vi "Drive Controller.vi"(8 "error in":errorcluster) -> ()   [LabVIEW 2020]
doc: "This VI executes continuously carrying out the current operation and responding to updates or new operation requests. It will often contain the timing or control code that is difficult to place directly in TeleOp. This VI generally opens all sensors and motors and isolates the rest of the robot code from knowing implementation details of how the operations are carried out."
uses:
  <vilib>/Rock Robotics/WPI/Framework/Completion Status.ctl
  Drive Setpoints.ctl
  Drive Operations.ctl
  <vilib>/Rock Robotics/WPI/SafetyOutput/WPI_SafetyOutputConfigMenu.ctl
  <vilib>/Rock Robotics/WPI/ThirdParty/REV Robotics/REVLib/Typedef/Spark MAX Idle Mode.ctl
  <vilib>/Rock Robotics/WPI/RobotDrive/WPI_RobotDriveOpen2MotorWithExistingMotors.vi
  <vilib>/Rock Robotics/Network Tables/NT Write Numeric Array.vi
  <vilib>/Rock Robotics/WPI/ThirdParty/REV Robotics/REVLib/Typedef/Spark MAX Motor Type.ctl
panel:
  in  "Interactive Values":T1
  in  "Buttons":cluster{"Execute Cmd":bool, "Abort Cmd":bool}
  out "Command Timing":cluster{"Start Time (ms)":u32, "Iterations":i32}
  out "Status":T3
  out "Setpoints":T4(graph)
  out "Current\nCmd":string
  # "Tip: The graph shows the motor setpoints. It may also be helpful to observe inputs and sensor values.\nYou may also want to display tuning or debugging controls."
  # "Interactive Command: You may fill in the settings for a command\nand schedule it with the Execute button. You can observe and abort\nany command while fine tuning the code for the controller."
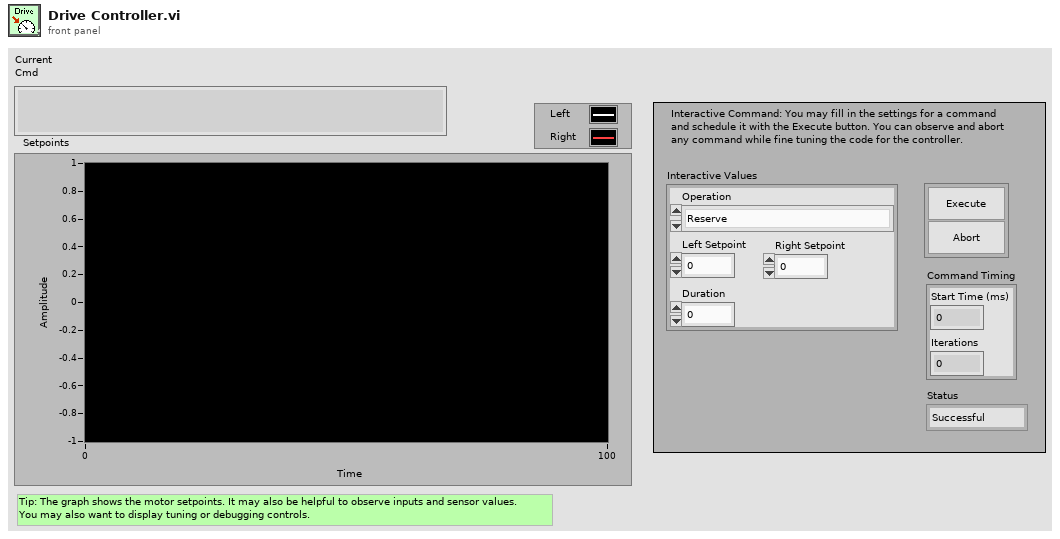
[diagram p1: front panel]
types:
  T1 = typedef "Drive Setpoints.ctl" = cluster{"Operation":T2, "Left Setpoint":dbl, "Right Setpoint":dbl, "Duration":dbl}
  T2 = typedef "Drive Operations.ctl" = enum16{"Reserve", "Read Current", "Immediate", "Drive for Time", "Drive for Distance"}
  T3 = typedef "Completion Status.ctl" = enum16{"Successful", "Aborted", "Incomplete"}
  T4 = cluster{"Left Setpoint":dbl, "Right Setpoint":dbl}
  T5 = typedef "WPI_SafetyOutputConfigMenu.ctl" = enum16{"Enable", "Disable"}
  T6 = typedef "Spark MAX Idle Mode.ctl" = enum16{"Coast", "Brake"}
  T7 = typedef "WPI_MotorControlDeviceRef.ctl" = cluster{"DeviceStatus":errorcluster, "Type":T8, "PWM":cluster{"PWM Channel":T9, "DeadBand":T10}, "CAN":cluster{"Device Number":u8, "SetOutput VI Ref":variant, "GetOutput VI Ref":variant, "Enable VI Ref":variant, "Disable VI Ref":variant, "Data":variant}, "Invert":bool, "DIO PWM":cluster{"PWM \"Enable\" Channel":T9, "DIOChannel":T11, "PWM Rate":dbl}}
  T8 = typedef "WPI_MotorControlType.ctl" = enum16{"PWM", "CAN", "DIO PWM"}
  T9 = typedef "FPGA_DIOPWMChannel.ctl" = enum8{"PWM 0", "PWM 1", "PWM 2", "PWM 3", "PWM 4", "PWM 5", "PWM 6", "PWM 7", "PWM 8", "PWM 9", "PWM MXP 0", "PWM MXP 1", "PWM MXP 2", "PWM MXP 3", "PWM MXP 4", "PWM MXP 5", "PWM MXP 6", "PWM MXP 7", "PWM MXP 8", "PWM MXP 9", "Invalid"}
  T10 = typedef "WPI_PWMDeadband.ctl" = cluster{"Name":string, "maxPositivePwm":i32, "minPositivePwm":i32, "centerPwm":i32, "maxNegativePwm":i32, "minNegativePwm":i32, "angularRange":u16}
  T11 = typedef "FPGA_DIOChannel.ctl" = enum8{"DIO 0", "DIO 1", "DIO 2", "DIO 3", "DIO 4", "DIO 5", "DIO 6", "DIO 7", "DIO 8", "DIO 9", "DIO MXP 0", "DIO MXP 1", "DIO MXP 2", "DIO MXP 3", "DIO MXP 4", "DIO MXP 5", "DIO MXP 6", "DIO MXP 7", "DIO MXP 8", "DIO MXP 9", "DIO MXP 10", "DIO MXP 11", "DIO MXP 12", "DIO MXP 13", "DIO MXP 14", "DIO MXP 15", "SPI Port CS1", "SPI Port CS2", "SPI Port CS3", "SPI Port MISO", "SPI Port MOSI", "Invalid"}
  T12 = typedef "Spark MAX Motor Type.ctl" = enum16{"Brushed", "Brushless"}
  T13 = typedef "WPI_RobotDriveDevRef.ctl" = cluster{"DevStatus":errorcluster, "Motors[]":T7[], "Square Inputs":bool, "Max Output":dbl}
  T14 = typedef "Command Status Info.ctl" = cluster{"Name":string, "Status":T3, "notifier out":T15}
  T15 = typedef "Completion Notifier.ctl" = refnum<notifier>
  T16 = cluster{"SubSystem Data":T1, cluster{"Start Time (ms)":u32, "Iterations":i32}, cluster{"Command Info":T14, "Description":string, "Default Command":T1, "queue out":refnum<queue>, "Subsystem Name":string}}
  T17 = cluster{"SubSystem Data":T1, cluster{"Start Time (ms)":u32, "Iterations":i32}, "Default Command Arguments":cluster{"Command Info":T14, "Description":string, "Default Command":T1, "queue out":refnum<queue>, "Subsystem Name":string}}
  T18 = cluster{"Don't move motors while reserved":dbl, "Don't move motors while reserved":dbl}
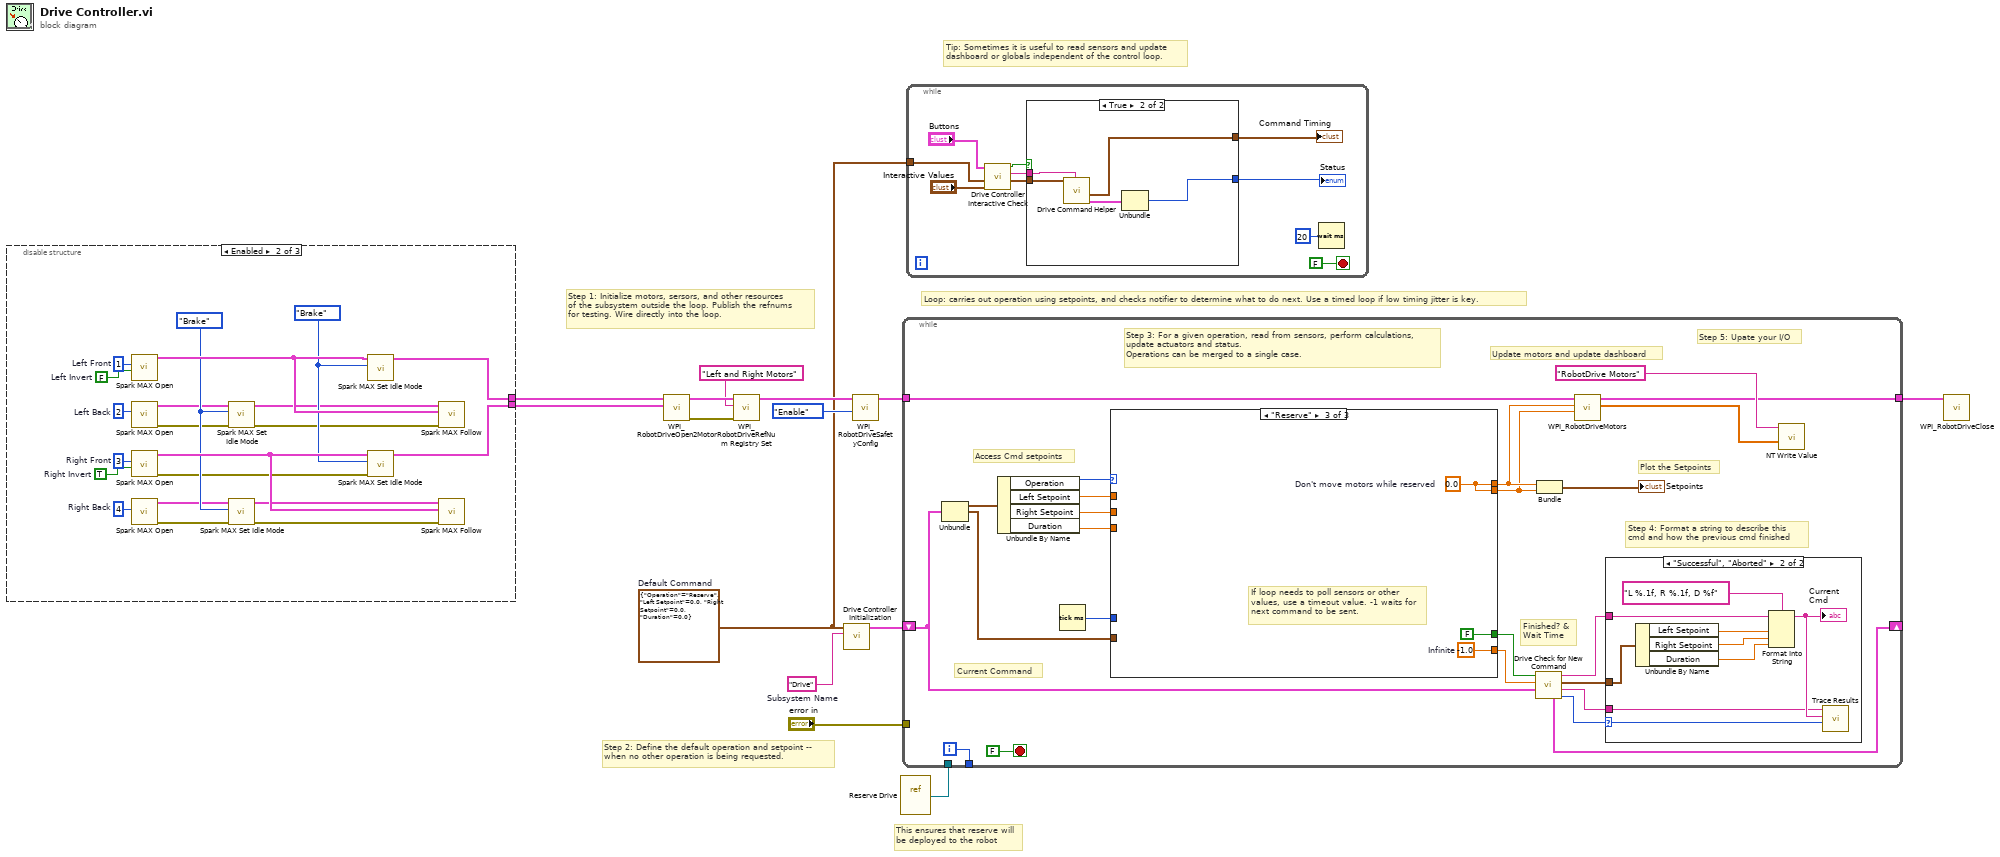
[diagram p0: block diagram]
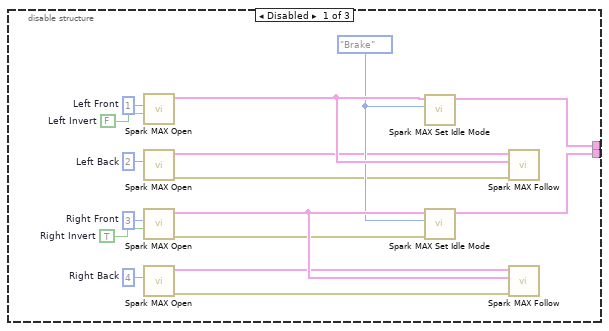
[diagram p2: hidden frame]
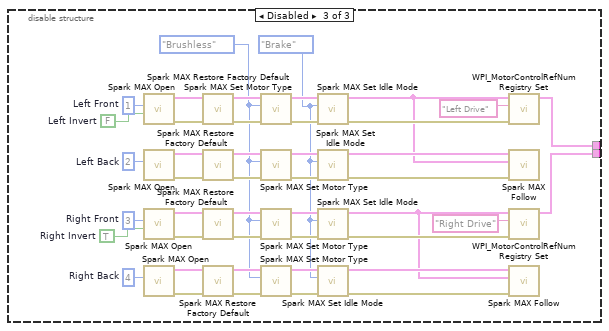
[diagram p3: hidden frame]
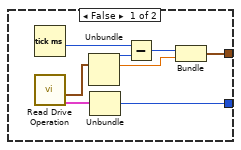
[diagram p4: hidden frame]
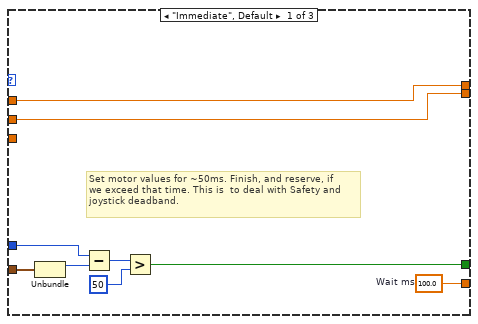
[diagram p6: hidden frame]
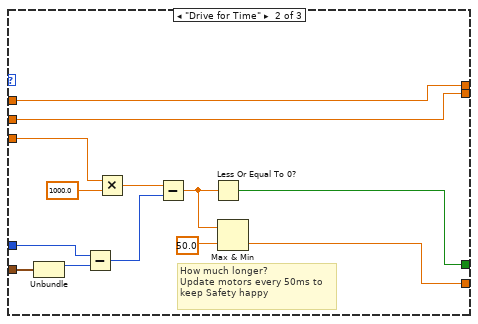
[diagram p7: hidden frame]
diagram:
  w4 = T1 {"Operation"=enum."Reserve", "Left Setpoint"=0.0, "Right Setpoint"=0.0, "Duration"=0.0}  # Default Command
  w14 = "Drive"  # Subsystem Name
  # "This ensures that reserve will\nbe deployed to the robot"
  # "Tip: Sometimes it is useful to read sensors and update\ndashboard or globals independent of the control loop."
  # "Step 2: Define the default operation and setpoint --\nwhen no other operation is being requested."
  # "Step 1: Initialize motors, sersors, and other resources\nof the subsystem outside the loop. Publish the refnums\nfor testing. Wire directly into the loop."
  # "Loop: carries out operation using setpoints, and checks notifier to determine what to do next. Use a timed loop if low timing jitter is key."
  n1 = disable-structure shown="Enabled" {
    disable-tunnel: [w23 w44 w55] -> w3
    disable-tunnel: [w21 w42 w54] -> w2
    frame Disabled {
      w20 = Spark_MAX_Idle_Mode."Brake" ("Idle Mode")
      w25 = u8 4  # Right Back
      w26 = u8 3  # Right Front
      w27 = u8 2  # Left Back
      w28 = u8 1  # Left Front
      w29 = TRUE  # Right Invert
      w30 = FALSE  # Left Invert
      n2 = call <vilib>:"Spark MAX Open.vi"("Invert"=w30, "Device Number"=w28) -> ("MotorControlDeviceRef"=w24:T7)  [unwired: 8 in, 1 out]
      n3 = call <vilib>:"Spark MAX Open.vi"("Device Number"=w27) -> ("error out"=w18:errorcluster, "MotorControlDeviceRef"=w19:T7)  [unwired: 9 in]
      n4 = call <vilib>:"Spark MAX Open.vi"("Invert"=w29, "Device Number"=w26) -> ("error out"=w17:errorcluster, "MotorControlDeviceRef"=w22:T7)  [unwired: 8 in]
      n5 = call <vilib>:"Spark MAX Open.vi"("Device Number"=w25) -> ("error out"=w15:errorcluster, "MotorControlDeviceRef"=w16:T7)  [unwired: 9 in]
      n6 = call <vilib>:"Spark MAX Set Idle Mode.vi"("Idle Mode"=w20, "MotorControlDeviceRef in"=w24) -> ("MotorControlDeviceRef out"=w23:T7)  [unwired: 8 in, 1 out]
      n7 = call <vilib>:"Spark MAX Set Idle Mode.vi"("error in (no error)"=w17, "Idle Mode"=w20, "MotorControlDeviceRef in"=w22) -> ("MotorControlDeviceRef out"=w21:T7)  [unwired: 7 in, 1 out]
      n8 = call <vilib>:"Spark MAX Follow.vi"("error in (no error)"=w18, "Master Controller"=w24, "MotorControlDeviceRef"=w19) -> ()  [unwired: 7 in, 2 out]
      n9 = call <vilib>:"Spark MAX Follow.vi"("error in (no error)"=w15, "Master Controller"=w22, "MotorControlDeviceRef"=w16) -> ()  [unwired: 7 in, 2 out]
    }
    frame Enabled {
      w40 = Spark_MAX_Idle_Mode."Brake" ("Idle Mode")
      w41 = Spark_MAX_Idle_Mode."Brake" ("Idle Mode")
      w46 = u8 4  # Right Back
      w47 = u8 3  # Right Front
      w48 = u8 2  # Left Back
      w49 = u8 1  # Left Front
      w50 = TRUE  # Right Invert
      w51 = FALSE  # Left Invert
      n10 = call <vilib>:"Spark MAX Open.vi"("Invert"=w51, "Device Number"=w49) -> ("MotorControlDeviceRef"=w45:T7)  [unwired: 8 in, 1 out]
      n11 = call <vilib>:"Spark MAX Open.vi"("Device Number"=w48) -> ("error out"=w37:errorcluster, "MotorControlDeviceRef"=w39:T7)  [unwired: 9 in]
      n12 = call <vilib>:"Spark MAX Open.vi"("Invert"=w50, "Device Number"=w47) -> ("error out"=w35:errorcluster, "MotorControlDeviceRef"=w43:T7)  [unwired: 8 in]
      n13 = call <vilib>:"Spark MAX Open.vi"("Device Number"=w46) -> ("error out"=w32:errorcluster, "MotorControlDeviceRef"=w34:T7)  [unwired: 9 in]
      n14 = call <vilib>:"Spark MAX Set Idle Mode.vi"("error in (no error)"=w37, "Idle Mode"=w40, "MotorControlDeviceRef in"=w39) -> ("error out"=w36:errorcluster, "MotorControlDeviceRef out"=w38:T7)  [unwired: 7 in]
      n15 = call <vilib>:"Spark MAX Set Idle Mode.vi"("error in (no error)"=w32, "Idle Mode"=w40, "MotorControlDeviceRef in"=w34) -> ("error out"=w31:errorcluster, "MotorControlDeviceRef out"=w33:T7)  [unwired: 7 in]
      n16 = call <vilib>:"Spark MAX Set Idle Mode.vi"("Idle Mode"=w41, "MotorControlDeviceRef in"=w45) -> ("MotorControlDeviceRef out"=w44:T7)  [unwired: 8 in, 1 out]
      n17 = call <vilib>:"Spark MAX Set Idle Mode.vi"("error in (no error)"=w35, "Idle Mode"=w41, "MotorControlDeviceRef in"=w43) -> ("MotorControlDeviceRef out"=w42:T7)  [unwired: 7 in, 1 out]
      n18 = call <vilib>:"Spark MAX Follow.vi"("error in (no error)"=w36, "Master Controller"=w45, "MotorControlDeviceRef"=w38) -> ()  [unwired: 7 in, 2 out]
      n19 = call <vilib>:"Spark MAX Follow.vi"("error in (no error)"=w31, "Master Controller"=w43, "MotorControlDeviceRef"=w33) -> ()  [unwired: 7 in, 2 out]
    }
    frame Disabled {
      w52 = Spark_MAX_Idle_Mode."Brake" ("Idle Mode")
      w53 = Spark_MAX_Motor_Type."Brushless" ("Motor Type")
      w62 = u8 4  # Right Back
      w63 = u8 3  # Right Front
      w64 = u8 2  # Left Back
      w65 = u8 1  # Left Front
      w66 = TRUE  # Right Invert
      w67 = FALSE  # Left Invert
      n20 = call <vilib>:"Spark MAX Open.vi"("Invert"=w67, "Device Number"=w65) -> ("error out"=w95:errorcluster, "MotorControlDeviceRef"=w94:T7)  [unwired: 8 in]
      n21 = call <vilib>:"Spark MAX Open.vi"("Device Number"=w64) -> ("error out"=w84:errorcluster, "MotorControlDeviceRef"=w85:T7)  [unwired: 9 in]
      n22 = call <vilib>:"Spark MAX Open.vi"("Invert"=w66, "Device Number"=w63) -> ("error out"=w78:errorcluster, "MotorControlDeviceRef"=w79:T7)  [unwired: 8 in]
      n23 = call <vilib>:"Spark MAX Open.vi"("Device Number"=w62) -> ("error out"=w73:errorcluster, "MotorControlDeviceRef"=w72:T7)  [unwired: 9 in]
      n24 = call <vilib>:"Spark MAX Restore Factory Default.vi"("error in"=w95, "MotorControlDeviceRef"=w94) -> ("error out"=w93:errorcluster, "MotorControlDeviceRef"=w92:T7)  [unwired: 8 in]
      n25 = call <vilib>:"Spark MAX Restore Factory Default.vi"("error in"=w84, "MotorControlDeviceRef"=w85) -> ("error out"=w86:errorcluster, "MotorControlDeviceRef"=w87:T7)  [unwired: 8 in]
      n26 = call <vilib>:"Spark MAX Restore Factory Default.vi"("error in"=w78, "MotorControlDeviceRef"=w79) -> ("error out"=w80:errorcluster, "MotorControlDeviceRef"=w81:T7)  [unwired: 8 in]
      n27 = call <vilib>:"Spark MAX Restore Factory Default.vi"("error in"=w73, "MotorControlDeviceRef"=w72) -> ("error out"=w71:errorcluster, "MotorControlDeviceRef"=w70:T7)  [unwired: 8 in]
      n28 = call <vilib>:"Spark MAX Set Motor Type.vi"("error in (no error)"=w93, "Motor Type"=w53, "MotorControlDevRef"=w92) -> ("error out"=w91:errorcluster, "MotorControlDeviceRef"=w90:T7)  [unwired: 7 in]
      n29 = call <vilib>:"Spark MAX Set Motor Type.vi"("error in (no error)"=w86, "Motor Type"=w53, "MotorControlDevRef"=w87) -> ("error out"=w88:errorcluster, "MotorControlDeviceRef"=w89:T7)  [unwired: 7 in]
      n30 = call <vilib>:"Spark MAX Set Motor Type.vi"("error in (no error)"=w80, "Motor Type"=w53, "MotorControlDevRef"=w81) -> ("error out"=w82:errorcluster, "MotorControlDeviceRef"=w83:T7)  [unwired: 7 in]
      n31 = call <vilib>:"Spark MAX Set Motor Type.vi"("error in (no error)"=w71, "Motor Type"=w53, "MotorControlDevRef"=w70) -> ("error out"=w69:errorcluster, "MotorControlDeviceRef"=w68:T7)  [unwired: 7 in]
      n32 = call <vilib>:"Spark MAX Set Idle Mode.vi"("error in (no error)"=w91, "Idle Mode"=w52, "MotorControlDeviceRef in"=w90) -> ("error out"=w61:errorcluster, "MotorControlDeviceRef out"=w59:T7)  [unwired: 7 in]
      n33 = call <vilib>:"Spark MAX Set Idle Mode.vi"("error in (no error)"=w88, "Idle Mode"=w52, "MotorControlDeviceRef in"=w89) -> ("error out"=w77:errorcluster, "MotorControlDeviceRef out"=w76:T7)  [unwired: 7 in]
      n34 = call <vilib>:"Spark MAX Set Idle Mode.vi"("error in (no error)"=w82, "Idle Mode"=w52, "MotorControlDeviceRef in"=w83) -> ("error out"=w60:errorcluster, "MotorControlDeviceRef out"=w58:T7)  [unwired: 7 in]
      n35 = call <vilib>:"Spark MAX Set Idle Mode.vi"("error in (no error)"=w69, "Idle Mode"=w52, "MotorControlDeviceRef in"=w68) -> ("error out"=w74:errorcluster, "MotorControlDeviceRef out"=w75:T7)  [unwired: 7 in]
      n36 = call <vilib>:"WPI_MotorControlRefNum Registry Set.vi"("error in (no error)"=w61, "refnum name"="Left Drive", "MotorControlDevRef"=w59) -> ("MotorControlDevRef"=w55:T7)  [unwired: 7 in, 1 out]
      n37 = call <vilib>:"Spark MAX Follow.vi"("error in (no error)"=w77, "Master Controller"=w59, "MotorControlDeviceRef"=w76) -> ()  [unwired: 7 in, 2 out]
      n38 = call <vilib>:"WPI_MotorControlRefNum Registry Set.vi"("error in (no error)"=w60, "refnum name"="Right Drive", "MotorControlDevRef"=w58) -> ("MotorControlDevRef"=w54:T7)  [unwired: 7 in, 1 out]
      n39 = call <vilib>:"Spark MAX Follow.vi"("error in (no error)"=w74, "Master Controller"=w58, "MotorControlDeviceRef"=w75) -> ()  [unwired: 7 in, 2 out]
    }
  }
  n40 = call-poly <vilib>:"WPI_RobotDriveOpen2Motor.vi"("Right Motor Dev Ref"=w2, "Left Motor Dev Ref"=w3) -> ("error out"=w11:errorcluster, "RobotDriveDevRef"=w13:T13)  [unwired: 3 in, 5 out]
  n41 = call <vilib>:"WPI_RobotDriveRefNum Registry Set.vi"("error in (no error)"=w11, "refnum name"="Left and Right Motors", "RobotDriveDevRef"=w13) -> ("RobotDriveDevRef"=w10:T13)  [unwired: 1 in, 7 out]
  n42 = call "Drive Controller Initialization.vi"("Subsystem Name"=w14, "Default Command"=w4) -> ("Current Command"=w6:T16)  [unwired: 9 in]
  n43 = call <vilib>:"WPI_RobotDriveSafetyConfig.vi"("mode"=WPI_SafetyOutputConfigMenu."Enable", "RobotDriveDevRef"=w10) -> ("RobotDriveDevRef"=w8:T13)  [unwired: 8 in, 1 out]
  n44 = vi-ref "Reserve Drive.vi"() -> (w5:refnum<vi>)
  n45 = while {
    shift-right: [w106] -> _
    shift-left: w6 -> [w99]
    tunnel: [w118] -> _
    tunnel: w8 -> [w114]
    tunnel: "error in" -> [_]
    tunnel: w5 -> [_]
    tunnel: [w96] -> w1
    i -> [w118]
    stop <- FALSE stop-if-true
    # "Step 5: Upate your I/O"
    # "Step 4: Format a string to describe this\ncmd and how the previous cmd finished"
    # "Current Command"
    # "Update motors and update dashboard"
    # "Plot the Setpoints"
    # "Access Cmd setpoints"
    # "Finished? &\nWait Time"
    # "Step 3: For a given operation, read from sensors, perform calculations,\nupdate actuators and status.\nOperations can be merged to a single case."
    n46 = Unbundle(w99) -> ("SubSystem Data"=w113:T1, w100:cluster{"Start Time (ms)":u32, "Iterations":i32})  [unwired: 1 out]
    n47 = Unbundle By Name(w113) -> ("Operation"=w112:T2, "Left Setpoint"=w111:dbl, "Right Setpoint"=w110:dbl, "Duration"=w109:dbl)
    n48 = Tick Count (ms)() -> (millisecond timer value=w108:u32)
    n49 = case shown="\"Reserve\"" w112 {
      tunnel: [w137 w138 w153] -> w105
      tunnel: [w130 w145 FALSE ("ignore previous (F)")] -> w104
      tunnel: w100 -> [w129 w147 _]
      tunnel: [w136 w144 w151] -> w116
      tunnel: [w135 w143 w151] -> w115
      tunnel: w111 -> [w136 w144 _]
      tunnel: w110 -> [w135 w143 _]
      tunnel: w109 -> [_ w142 _]
      tunnel: w108 -> [w131 w141 _]
      frame "Immediate", Default {
        w137 = 100.0  # Wait ms
        # "Set motor values for ~50ms. Finish, and reserve, if\nwe exceed that time. This is  to deal with Safety and\njoystick deadband."
        n50 = Unbundle(w129) -> ("Start Time (ms)"=w132:u32)  [unwired: 1 out]
        n51 = Subtract(x=w131, y=w132) -> (x-y=w133:u32)
        n52 = Greater?(x=w133, y=u8 50 ("Left Motor")) -> (0:w130:bool)
      }
      frame "Drive for Time" {
        # "How much longer?\nUpdate motors every 50ms to\nkeep Safety happy"
        n53 = Unbundle(w147) -> ("Start Time (ms)"=w146:u32)  [unwired: 1 out]
        n54 = Subtract(x=w141, y=w146) -> (x-y=w150:u32)
        n55 = Multiply(x=w142, y=1000.0) -> (x*y=w149:dbl)
        n56 = Subtract(x=w149, y=w150) -> (x-y=w140:dbl)
        n57 = Less Or Equal To 0?(x=w140) -> (x <= 0?=w145:bool)
        n58 = Max & Min(x=w140, y=50.0) -> (min(x,y)=w138:dbl)  [unwired: 1 out]
      }
      frame "Reserve" {
        w151 = 0.0  # Don't move motors while reserved
        w153 = -1.0  # Infinite
        # "If loop needs to poll sensors or other\nvalues, use a timeout value. -1 waits for\nnext command to be sent."
      }
    }
    n59 = call "Drive Check for New Command.vi"("input cluster"=w99, "Wait time (ms)"=w105, "Finished?"=w104) -> ("Completion"=w107:T3, "Subsystem Name"=w101:string, "Current Command"=w102:T1, "Initial Trace String"=w103:string, "Next Command"=w106:T17)  [unwired: 4 in]
    n60 = Bundle("Don't move motors while reserved"=w116, "Don't move motors while reserved"=w115) -> (→"Setpoints":T18)  [unwired: 1 in]
    n61 = call <vilib>:"WPI_RobotDriveMotors.vi"("RightSpeed"=w115, "LeftSpeed"=w116, "RobotDriveDevRef"=w114) -> ("Motor Values"=w97:dbl[], "RobotDriveDevRef"=w96:T13)  [unwired: 1 in, 6 out]
    n62 = case shown="\"Successful\", \"Aborted\"" w107 {
      selector: w107 -> [_ w128]
      tunnel: w103 -> [_ w123]
      tunnel: w102 -> [_ w124]
      tunnel: w101 -> [_ w120]
      frame "Incomplete", Default {
        # "Continuing current command"
      }
      frame "Successful", "Aborted" {
        # "Report and setup for next command"
        n63 = Unbundle By Name(w124) -> ("Left Setpoint"=w126:dbl, "Right Setpoint"=w127:dbl, "Duration"=w121:dbl)
        n64 = Format Into String(format string="L %.1f, R %.1f, D %f", initial string=w123, w126, w127, w121) -> (resulting string=w122:string)  [unwired: 1 in, 1 out]
        "Current\nCmd" <- w122
        n65 = call <vilib>:"Trace Results.vi"("Status of previous command"=w128, "Description"=w122, "Subsystem"=w120) -> ()  [unwired: 9 in]
      }
    }
    n66 = call-poly <vilib>:"NT Write Value.vi"("Numeric Array"=w97, "Name"="RobotDrive Motors") -> ()  [unwired: 9 in, 1 out]
  }
  n67 = while {
    tunnel: w4 -> [w155]
    stop <- FALSE stop-if-true
    n68 = call "Drive Controller Interactive Check.vi"("Interactive Command In"="Interactive Values", "Default Command"=w155, "Buttons"="Buttons") -> ("Interactive Command Out"=w157:T1, "Trace String"=w158:string, "Schedule"=w159:bool)  [unwired: 6 in]
    n69 = case shown="True" w159 {
      tunnel: [w168 w176] -> w160
      tunnel: [w167 w172] -> w161
      tunnel: w158 -> [_ w174]
      tunnel: w157 -> [_ w173]
      frame False {
        n70 = Tick Count (ms)() -> (millisecond timer value=w171:u32)
        n71 = call "Read Drive Operation.vi"() -> ("Command Info"=w165:T14, "SubSystem Data"=w164:T1)  [unwired: 9 in, 1 out]
        n72 = Unbundle(w164) -> ("Operation"=w169:T2, "Left Setpoint"=w166:dbl)  [unwired: 2 out]
        n73 = Unbundle(w165) -> ("Status"=w168:T3)  [unwired: 2 out]
        n74 = Subtract(x=w171, y=w169) -> (x-y=w170:u32)
        n75 = Bundle(w170, "Left Setpoint"=w166) -> (w167:cluster{u32, "Left Setpoint":dbl})  [unwired: 1 in]
      }
      frame True {
        n76 = call "Drive Command Helper.vi"("Description"=w174, "SubSystem Data"=w173) -> ("Command Info Out"=w175:T14, "Command Timing"=w172:cluster{"Start Time (ms)":u32, "Iterations":i32})  [unwired: 7 in, 1 out]
        n77 = Unbundle(w175) -> ("Status"=w176:T3)  [unwired: 2 out]
      }
    }
    "Status" <- w160
    "Command Timing" <- w161
    n78 = Wait (ms)(milliseconds to wait=u32 20) -> ()  [unwired: 1 out]
  }
  n79 = call <vilib>:"WPI_RobotDriveClose.vi"("RobotDriveDevRef"=w1) -> ()  [unwired: 10 in, 1 out]
